vi "Write TestResultInformation.vi"(8 "error in (no error)":errorcluster, 10 "TestResultInformation":T1, 11 "TestBench in":refnum<class "TestBench.lvclass">) -> (0 "error out":errorcluster, 3 "TestBench out":refnum<class "TestBench.lvclass">)   [LabVIEW 2019, in "TestBench.lvlib" / "TestBench.lvclass"]
uses:
  TestBench.lvclass
  TestBench.lvclass/TestBench.ctl
  LocalReport/LocalReport Messages/SaveReport Msg/SaveReport Msg.lvclass/SaveReport Msg.ctl
  <vilib>/ActorFramework/Message Enqueuer/Message Enqueuer.lvclass/Message Enqueuer.ctl
  SignalProcessing/SignalProcessing Messages/TestComplete Msg/TestComplete Msg.lvclass/TestComplete Msg.ctl
  968f84f9-fca7-492d-bcae-7387758258c9.vi
  <vilib>/ActorFramework/Message Enqueuer/Enqueue.vi
  LocalReport/LocalReport Messages/SaveReport Msg/SaveReport Msg.lvclass
  C:/Program Files (x86)/National Instruments/LabVIEW 2019/vi.lib/ActorFramework/Message/Message.lvclass
  SignalProcessing/SignalProcessing Messages/TestComplete Msg/TestComplete Msg.lvclass
  <vilib>/ActorFramework/Message Priority Queue/Priority Enqueue.vi
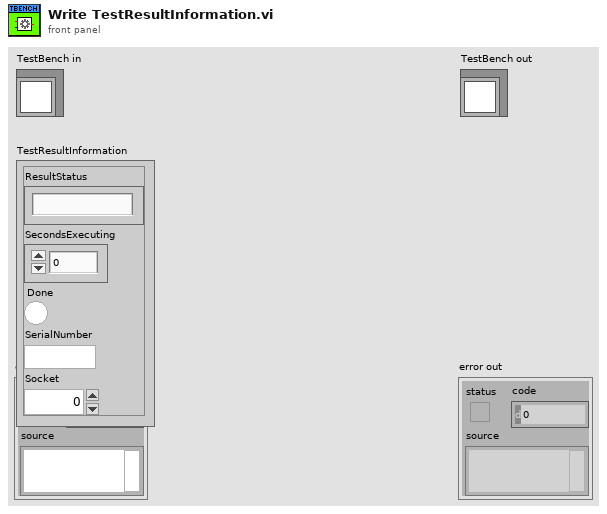
[diagram p1: front panel]
types:
  T1 = cluster{"ResultStatus":string, "SecondsExecuting":dbl, "Done":bool, "SerialNumber":string, "Socket":i32}
  T2 = enum8{"Enabled", "Disabled", "Disabled and Grayed Out"}
  T3 = cluster{"2D Picture":picture, "Pass":u32, "Fail":u32, "Yield":dbl, "Total":u32}
  T4 = cluster{"ResultStatus":string, "SecondsExecuting":dbl, "SerialNumber":string, "Value":string}
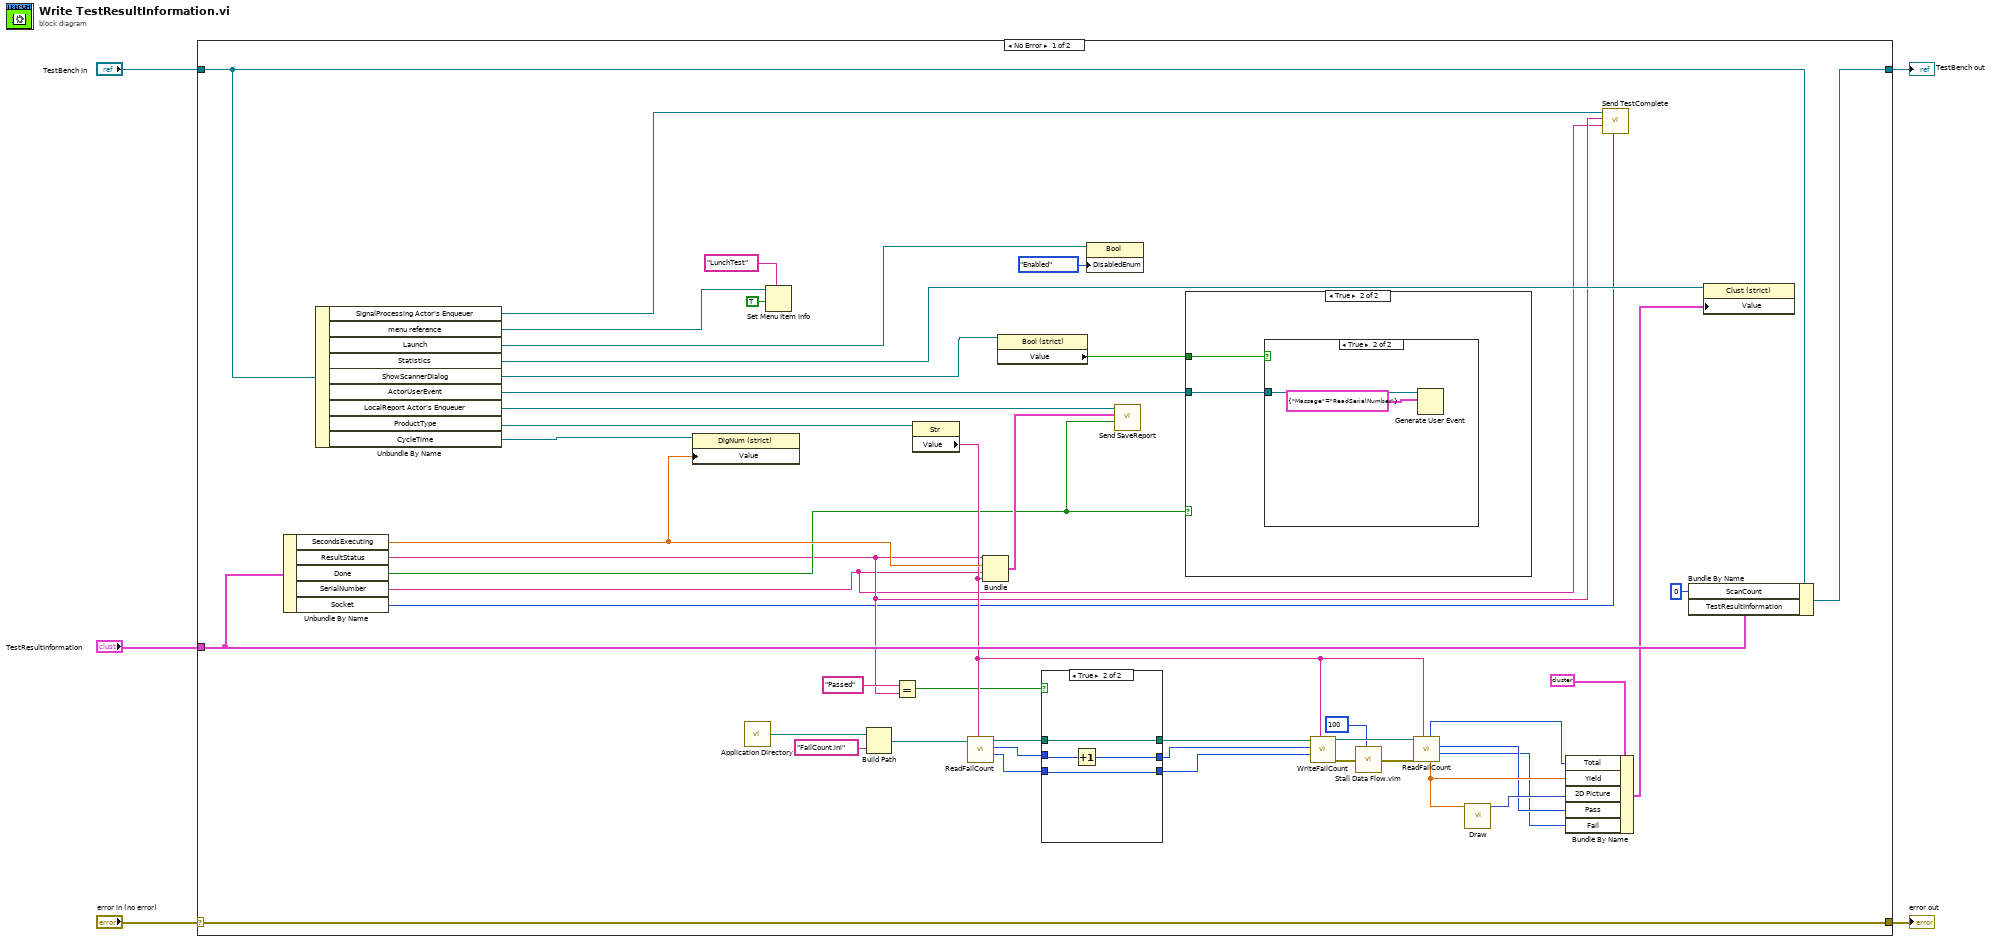
[diagram p0: block diagram]
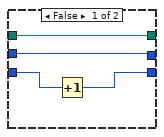
[diagram p4: hidden frame]
diagram:
  n1 = case shown="No Error" "error in (no error)" {
    selector: "error in (no error)" -> [w52 w65]
    tunnel: [w52 w65] -> w4
    tunnel: [w51 w66] -> w2
    tunnel: "TestBench in" -> [w49 w66]
    tunnel: "TestResultInformation" -> [w50 _]
    frame No Error {
      n2 = Unbundle By Name(w50) -> ("SecondsExecuting"=w47:dbl, "ResultStatus"=w8:string, "Done"=w9:bool, "SerialNumber"=w7:string, "Socket"=w6:i32)
      n3 = Unbundle By Name(w49) -> ("SignalProcessing Actor's Enqueuer"=w13:refnum<class "Message Enqueuer.lvclass">, "menu reference"=w14:refnum<k9>, "Launch"=w18:refnum<vi>, "Statistics"=w32:refnum<vi>, "ShowScannerDialog"=w44:refnum<vi>, "ActorUserEvent"=w45:refnum<user-event>, "LocalReport Actor's Enqueuer"=w11:refnum<class "Message Enqueuer.lvclass">, "ProductType"=w46:refnum<vi>, "CycleTime"=w48:refnum<vi>)
      n4 = property class="DigNum (strict)"(reference=w48, "Value"=w47) -> ()  [unwired: 1 in, 2 out]
      n5 = call <vilib>:"Application Directory.vi"() -> ("Application Directory"=w41:path)
      n6 = Set Menu Item Info(7:"LunchTest" ("item tag"), 9:TRUE ("enabled"), 11:w14) -> ()  [unwired: 4 in, 2 out]
      n7 = Build Path(base path=w41, name or relative path="FailCount.ini") -> (appended path=w39:path)
      n8 = Equal?(x="Passed" ("y"), y=w8) -> (x = y?=w12:bool)
      n9 = property class="Str"(reference=w46) -> ("Value"=w31:string)  [unwired: 1 in, 2 out]
      n10 = call "ReadFailCount.vi"("ProductModle"=w31, "Statistics path"=w39) -> ("Fail"=w36:u32, "Pass"=w37:u32, "file path"=w38:path)  [unwired: 4 in, 3 out]
      n11 = Bundle("ResultStatus"=w8, "SecondsExecuting"=w47, "SerialNumber"=w7, "Value"=w31) -> (w10:T4)  [unwired: 1 in]
      n12 = property class="Bool (strict)"(reference=w44) -> ("Value"=w43:bool)  [unwired: 1 in, 2 out]
      n13 = case shown="True" w12 {
        tunnel: w37 -> [w60 w64]
        tunnel: [w60 w63] -> w34
        tunnel: w36 -> [w59 w62]
        tunnel: [w58 w62] -> w33
        tunnel: w38 -> [w57 w61]
        tunnel: [w57 w61] -> w35
        frame False {
          n14 = Increment(x=w59) -> (x+1=w58:u32)
        }
        frame True {
          n15 = Increment(x=w64) -> (x+1=w63:u32)
        }
      }
      n16 = property class="Bool"(reference=w18, "DisabledEnum"=T2."Enabled" ("Disabled")) -> ()  [unwired: 1 in, 2 out]
      n17 = call "Send SaveReport.vi"("Done"=w9, "TestResultInformation"=w10, "Message Enqueuer"=w11) -> ()  [unwired: 7 in, 2 out]
      n18 = case shown="True" w9 {
        tunnel: w45 -> [_ w54]
        tunnel: w43 -> [_ w53]
        frame False {
        }
        frame True {
          n19 = case shown="True" w53 {
            tunnel: w54 -> [_ w56]
            frame False {
            }
            frame True {
              n20 = Generate User Event(user event=w56, event data cluster=cluster{"Massage":string} {"Massage"="ReadSerialNumber"} ("event data")) -> ()  [unwired: 2 in, 2 out]
            }
          }
        }
      }
      n21 = call "WriteFailCount.vi"("SequenceFillePath"=w31, "Fail"=w33, "Pass"=w34, "Statistics path"=w35) -> ("error out"=w29:errorcluster, "file path"=w30:path)  [unwired: 6 in]
      n22 = call "Stall Data Flow.vim"("value in"=w29, "milliseconds to wait"=u32 100) -> ("value out"=w28:errorcluster)  [unwired: 1 out]
      n23 = call "ReadFailCount.vi"("ProductModle"=w31, "error in (no error)"=w28, "Statistics path"=w30) -> ("Fail"=w22:u32, "Pass"=w23:u32, "yield"=w25:dbl, "Total"=w21:u32)  [unwired: 3 in, 2 out]
      n24 = call "Draw.vi"("Yeld"=w25) -> ("2D Picture"=w24:picture)  [unwired: 10 in]
      n25 = Bundle By Name(cluster=T3 {"2D Picture"=bytes[0], "Pass"=0, "Fail"=0, "Yield"=0.0, "Total"=0} ("Value"), "Total"=w21, "Yield"=w25, "2D Picture"=w24, "Pass"=w23, "Fail"=w22) -> (w20:T3)
      n26 = call "Send TestComplete.vi"("Socket"=w6, "SerialNumber"=w7, "TestResult"=w8, "Message Enqueuer"=w13) -> ()  [unwired: 6 in, 2 out]
      n27 = Bundle By Name(cluster=w49, "ScanCount"=u8 0, "TestResultInformation"=w50) -> (w51:refnum<class "TestBench.lvclass">)
      n28 = property class="Clust (strict)"(reference=w32, "Value"=w20) -> ()  [unwired: 1 in, 2 out]
    }
    frame Error {
    }
  }
  "error out" <- w4
  "TestBench out" <- w2
